vi "ukol3.vi"() -> ()   [LabVIEW 2023]
uses:
  <vilib>/measure/NI_MABase.lvlib
  <vilib>/gmath/NI_Gmath.lvlib
panel:
  out "size(s)":i32
  out "error":i32
  out "Waveform Graph 2":waveform(dbl)[](graph)
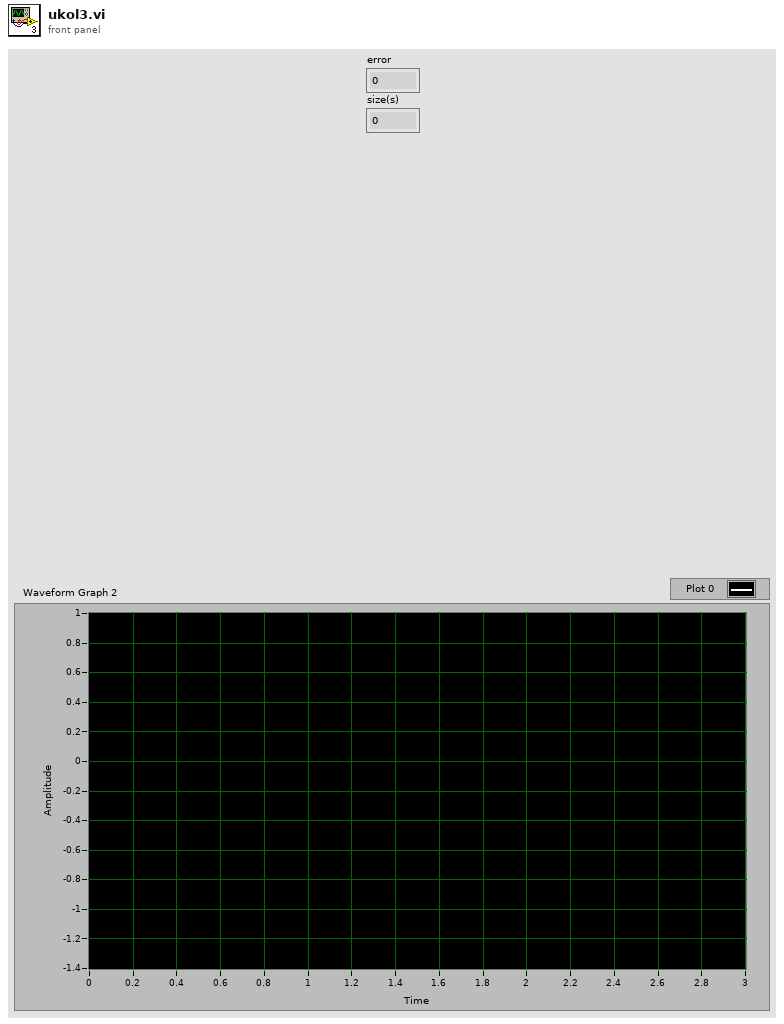
[diagram p1: front panel]
types:
  T1 = cluster{"frequency":dbl, "amplitude":dbl, "phase":dbl}[]
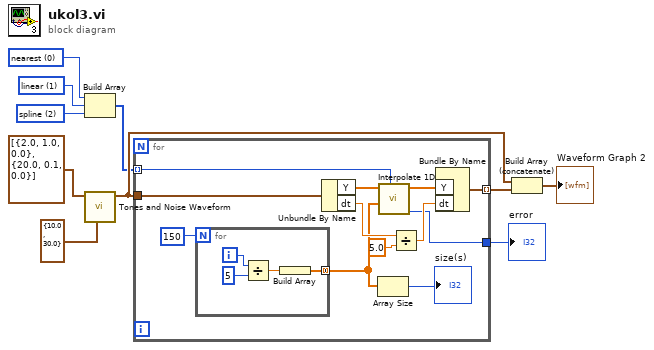
[diagram p0: block diagram]
diagram:
  w5 = 2 items=["nearest", "linear", "spline", "cubic Hermite", "Lagrange"] ("method")
  w7 = 1 items=["nearest", "linear", "spline", "cubic Hermite", "Lagrange"] ("method")
  w6 = 0 items=["nearest", "linear", "spline", "cubic Hermite", "Lagrange"] ("method")
  n1 = Build Array(w6, w7, w5) -> (w3:i32[])
  n2 = call <vilib>:"Tones and Noise Waveform.vi"("sampling info"=cluster{"Fs":dbl, "#s":dbl} {"Fs"=10.0, "#s"=30.0}, "tones"=T1 [{"frequency"=2.0, "amplitude"=1.0, "phase"=0.0}, {"frequency"=20.0, "amplitude"=0.1, "phase"=0.0}]) -> ("signal out"=w4:waveform(dbl))  [unwired: 8 in, 1 out]
  n3 = for {
    tunnel: w4 -> [w18]
    tunnel: w3 -> [w17] mode=indexing
    tunnel: [w16] -> w2 mode=indexing
    tunnel: [w15] -> w1
    n4 = for {
      N: 150 -> [_]
      tunnel: [w23] -> w12 mode=concatenating
      i -> [w25]
      n5 = Divide(x=w25, y=5) -> (x/y=w26:dbl)
      n6 = Build Array(w26) -> (w23:dbl[])
    }
    n7 = Unbundle By Name(w18) -> ("Y"=w14:dbl[], "dt"=w21:dbl)
    n8 = Array Size(array=w12) -> (size(s)=→"size(s)":i32)
    n9 = call <vilib>:"Interpolate 1D.vi"("method"=w17, "xi"=w12, "Y"=w14) -> ("error"=w15:i32, "yi"=w20:dbl[])  [unwired: 6 in, 1 out]
    n10 = Divide(x=w21, y=5.0) -> (x/y=w22:dbl)
    n11 = Bundle By Name("Y"=w20, "dt"=w22) -> (w16:waveform(dbl))  [unwired: 1 in]
  }
  "error" <- w1
  n12 = Build Array (concatenate)(w4, w2) -> (→"Waveform Graph 2":waveform(dbl)[])
